vi "Load Seq.vi"(8 "Error In":errorcluster, 10 "Seq file path":path=path "C:/Users/skkjh/OneDrive - Chroma ATE/Working Copy/Cobra Single/NI-9651 SoM RT/RT_Configuration file/Cobra Extra Settings.ini", 11 "Sequence in":refnum<class "Sequence.lvclass">) -> (0 "error out":errorcluster, 3 "Sequence out":refnum<class "Sequence.lvclass">)   [LabVIEW 2019, in "Sequence.lvlib" / "Sequence.lvclass"]
uses:
  Sequence.lvclass
  C:/Program Files (x86)/National Instruments/LabVIEW 2019/vi.lib/ActorFramework/Actor/Actor.lvclass
  <vilib>/ActorFramework/Actor/Actor.lvclass/Actor.ctl
  Sequence.lvclass/Sequence.ctl
  Sequence Messages/Sequence Msg/Sequence Msg.lvclass/Sequence Msg.ctl
  <vilib>/ActorFramework/Message Enqueuer/Message Enqueuer.lvclass/Message Enqueuer.ctl
  <vilib>/ActorFramework/Message Enqueuer/Enqueue.vi
  Sequence Messages/Sequence Msg/Sequence Msg.lvclass
  C:/Program Files (x86)/National Instruments/LabVIEW 2019/vi.lib/ActorFramework/Message/Message.lvclass
  <vilib>/Utility/config.llb/Read Key (I32).vi
  <vilib>/Utility/config.llb/Read Key (U32).vi
  <vilib>/Utility/config.llb/Read Key (String).vi
  <vilib>/ActorFramework/Message Priority Queue/Priority Enqueue.vi
  <vilib>/Utility/config.llb/NI_LVConfig.lvlib
  <vilib>/ActorFramework/Actor/Actor.lvclass
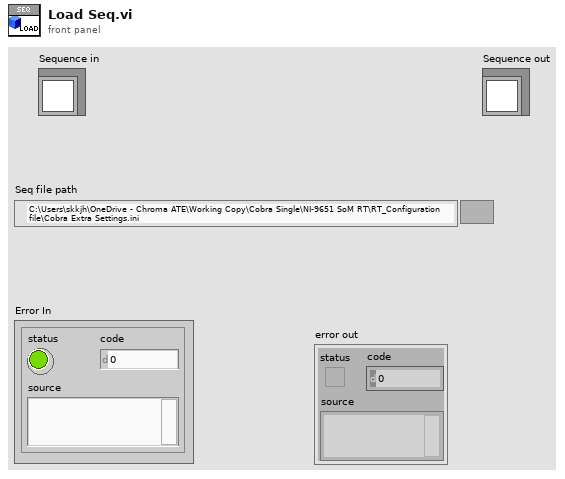
[diagram p1: front panel]
types:
  T1 = typedef "NI_LVConfig.lvlib/Config Data RefNum.ctl" = refnum<k1>
  T2 = cluster{"Duration":i32, "Value":u32, "Name":string}
  T3 = cluster{"Duration":i32, "Value":u32, "Name":string}[]
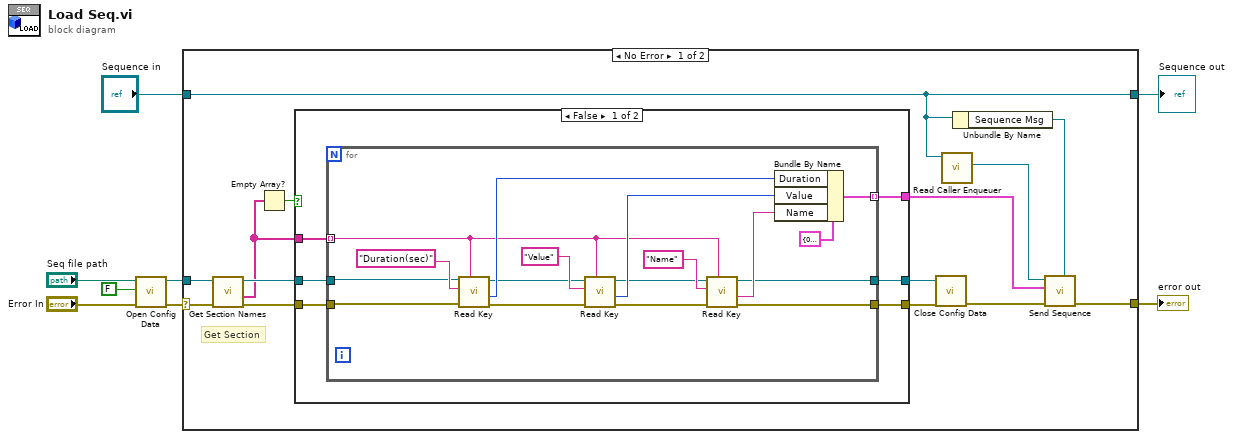
[diagram p0: block diagram]
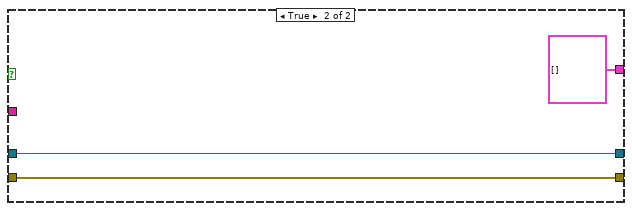
[diagram p2: hidden frame]
diagram:
  n1 = call <vilib>:"Open Config Data.vi"("error in (no error)"="Error In", "create file if necessary (T)"=FALSE, "configuration file path"="Seq file path") -> ("error out"=w2:errorcluster, "refnum"=w3:T1)  [unwired: 6 in, 1 out]
  n2 = case shown="No Error" w2 {
    selector: w2 -> [w20 w50]
    tunnel: [w11 w50] -> w8
    tunnel: [w10 w49] -> w6
    tunnel: "Sequence in" -> [w10 w49]
    tunnel: w3 -> [w18 _]
    frame No Error {
      # "Get Section"
      n3 = call <vilib>:"Get Section Names.vi"("error in (no error)"=w20, "refnum"=w18) -> ("error out"=w21:errorcluster, "section names"=w16:string[], "refnum out"=w22:T1)  [unwired: 7 in]
      n4 = Empty Array?(array=w16) -> (empty?=w15:bool)
      n5 = case shown="False" w15 {
        tunnel: w22 -> [w28 w48]
        tunnel: w21 -> [w27 w47]
        tunnel: [w26 w47] -> w19
        tunnel: [w25 w48] -> w17
        tunnel: [w24 T3 []] -> w13
        tunnel: w16 -> [w23 _]
        frame False {
          n6 = for {
            tunnel: w27 -> [w33]
            tunnel: w28 -> [w34]
            tunnel: w23 -> [w35] mode=indexing
            tunnel: [w37] -> w26
            tunnel: [w43] -> w24 mode=indexing
            tunnel: [w29] -> w25
            n7 = call-poly <vilib>:"Read Key.vi"("section"=w35, "error in (no error)"=w33, "key"="Duration(sec)", "refnum"=w34) -> ("error out"=w41:errorcluster, "value"=w44:i32, "refnum out"=w39:T1)  [unwired: 4 in, 1 out]
            n8 = call-poly <vilib>:"Read Key.vi"("section"=w35, "error in (no error)"=w41, "key"="Value", "refnum"=w39) -> ("error out"=w31:errorcluster, "value"=w40:u32, "refnum out"=w32:T1)  [unwired: 4 in, 1 out]
            n9 = call-poly <vilib>:"Read Key.vi"("section"=w35, "error in (no error)"=w31, "key"="Name", "refnum"=w32) -> ("error out"=w37:errorcluster, "value"=w36:string, "refnum out"=w29:T1)  [unwired: 4 in, 1 out]
            n10 = Bundle By Name(cluster=T2 {"Duration"=0, "Value"=0, "Name"=""} ("Sequence"), "Duration"=w44, "Value"=w40, "Name"=w36) -> (w43:T2)
          }
        }
        frame True {
        }
      }
      n11 = call <vilib>:"Close Config Data.vi"("error in (no error)"=w19, "refnum"=w17) -> ("error out"=w12:errorcluster)  [unwired: 8 in, 1 out]
      n12 = call <vilib>:"Read Caller Enqueuer.vi"("Actor"=w10) -> ("Caller Enqueuer"=w14:refnum<class "Message Enqueuer.lvclass">)  [unwired: 10 in]
      n13 = Unbundle By Name(w10) -> ("Sequence Msg"=w9:refnum<class "Sequence Msg.lvclass">)
      n14 = call "Send Sequence.vi"("Message Type"=w9, "error in (no error)"=w12, "Sequence"=w13, "Message Enqueuer"=w14) -> ("error out"=w11:errorcluster)  [unwired: 6 in, 1 out]
    }
    frame Error {
    }
  }
  "error out" <- w8
  "Sequence out" <- w6
